vi "DIC main 11082010.vi"() -> ()   [LabVIEW 2010]
panel:
  in  "pCO2_end":dbl
  in  "pCO2":dbl
  in  "pCO2_start":dbl
  in  "DataFile":path
  in  "sampleTime":dbl
  # "Global variables in Gernot's code:\nCO2pres\nCO2_Temp\nCom_Error\nCurrentRepeat\nDataFile\nError_Log\nH2O\nLicorData\nOperation\npCO2\npCO2_end\npCO2_integrate\npCO2_max\npCO2_start\nPeakAvg\nPeakRead\nRepeat\nSampleCount\nSampleID\nSampleTime\nSampleType\nSequenceTime\nSyringeCom\nTCO2Error\nValvePosition\nXplot\nYplot"
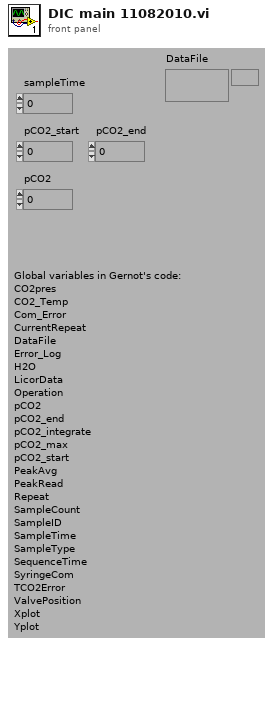
[diagram p1: front panel]
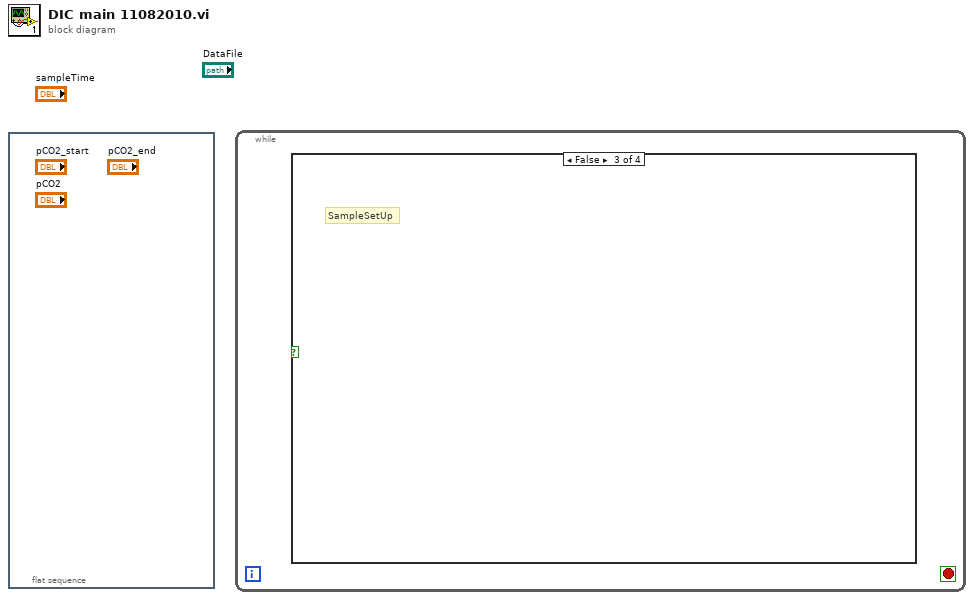
[diagram p0: block diagram]
diagram:
  n1 = flat-sequence {
    frame #0 {
    }
  }
  n2 = while {
    stop <- _ stop-if-true
    n3 = case shown="\"RunSample\"" {
      selector: _ -> [_ _ _ _]
      frame False {
      }
      frame True {
        # "note says: close dump then stop gas flow"
        # "Call stopGasFlow"
        # "Wait 1 seconds"
        # "Call Close Dump"
        # "Wait 5 seconds"
        # "init_Licor"
        # "Initialize Syringe"
        # "Open Dump"
      }
      frame False {
        # "SampleSetUp"
      }
      frame True {
        # "create a file to save data... give it a name with date and time"
      }
    }
  }
